vi "GoopDebugger.vi"(1 "ClassToOpen":string, 5 "error in (no error)":errorcluster) -> (19 "error out":errorcluster)   [LabVIEW 2020]
uses:
  <resource>/Framework/Providers/Open_GDS/SubVIs/GOOP_HelpButton.ctl
  <resource>/Framework/Providers/Open_GDS/ClassProviders/Common/LvClass_class/GDSLvClass_ProviderTypes.ctl
  <vilib>/Utility/miscctls.llb/LVRectTypeDef.ctl
  <resource>/Framework/Providers/Open_GDS/ClassProviders/Provider_EndevoGOOP300/ClassWriterGOOP300_class/ClassWriterGOOP300.lvclass
panel:
  in  "_GOOP4Control":bool
  in  "_Help":bool
  in  "_HelpDebugger":T1
  in  "_AttributeType":bool
  in  "_Classes":u16(ring) caption="Classes" items=["View all objects", "-", "GA.lvclass", "GB.lvclass", "GC.lvclass", "GD.lvclass", "File.lvclass", "MyFile.lvclass", "-", "Refresh list"]
  in  "_KillObject":bool
  in  "SortName":bool
  in  "SortId":bool
  out "_NoOfObjects":i32 caption="No of objects"
  in  "_Objects":i32(listbox) caption="Objects"
  out "_Project":string caption="Project"
  in  "_KillAll":bool
  in  "Next":bool
  in  "Prev":bool
  out "AttributeType":string
  in  "_LockPanel":bool
  in  "Update":bool
  in  "_Action":T2(ring) caption="Action"
  out "_Size (kB)":dbl caption="Size (kB)" format="%#.1f"
  out "_Locked?":bool caption="Locked"
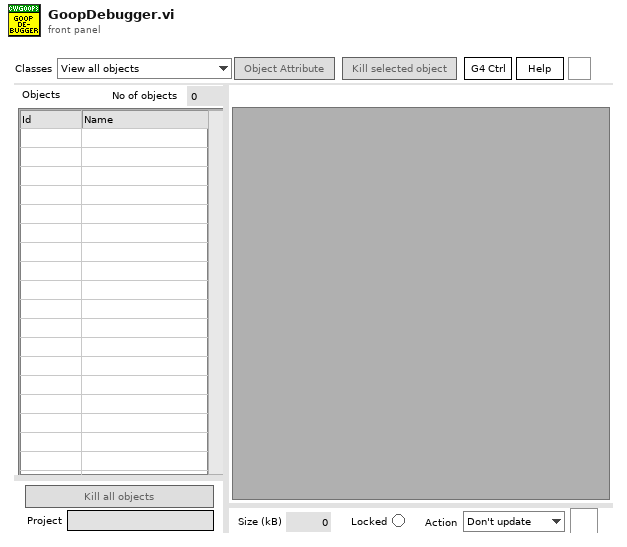
[diagram p1: front panel]
types:
  T1 = typedef "GOOP_HelpButton.ctl" = bool
  T2 = enum16{"Don't update", "Update once", "10ms", "100ms", "500ms", "1s", "2s", "Modify"}
  T3 = typedef "GDSLvClass_ProviderTypes.ctl" = enum16{"UnKnown(LabVOOP)", "Native", "EndevoGOOP3", "OpenG(RootObject)", "OpenG(OpenG_Object)", "EndevoGOOP4", "JKI1"}
  T4 = cluster{"Ref":i32, "Class":string, "Name":string, "ClassProvider":T3}[]
  T5 = typedef "LVRectTypeDef.ctl" = cluster{"Left":i16, "Top":i16, "Right":i16, "Bottom":i16}
  T6 = cluster{"Front Panel.WinBounds":T5, "FP.Behavior":enum32{"Invalid", "Default", "Floating", "Floating/Auto-Hide", "Modal"}}
  T7 = cluster{"DebugQueue":refnum<queue>, "Classes":string[], "ClassAttribute":bool, "NoClassesFound":bool, "ObjRefs":refnum<vi>[], "ClassAttRefs":refnum<vi>[], "ObjStatus":refnum<vi>[], "CurrentClassViewing":string, "ClassAttributeViewing":bool, "OldAction":enum16{"Don't update", "Update once", "10ms", "100ms", "500ms", "1s", "2s", "Modify"}, "ObjectAttString":string, "ClassAttString":string, "KillAllStr":string, "KillTheseStr":string, "IdSort":bool, "MyComputerRef":refnum<vi>, "ClassType":T3[], "ClRefs":refnum<vi>[], "ParentObjeRefs":refnum<vi>[], "G4GetObjStatusRef":refnum<vi>, "G4ParentClasses":string[], "G4AttLevel":i32, "G4NewAttribute":bool, "G4AttRefs":refnum<vi>, "Objects":cluster{"Refs":variant, "VI Name":string, "Object name":string, "ClassProvider":T3}[], "PrevoiusG4AttLevel":i32, "Application":refnum<vi>, "G4ClassAttRefs":refnum<vi>}
  T8 = enum32{"Invalid", "Default", "Floating", "Floating/Auto-Hide", "Modal"}
  T9 = cluster{"Refs":variant, "VI Name":string, "Object name":string, "ClassProvider":T3}[]
  T10 = enum8{"Enabled", "Disabled", "Disabled and Grayed Out"}
  T11 = cluster{"Object names":string[], "Refs":variant[], "ObjectAttributeLocked":bool, "ClassAttributeLocked":bool, "ObjAttribute":variant, "ClassAttribute":variant}
  T12 = cluster{"Refs":variant, "VI Name":string, "Object name":string, "ClassProvider":T3}
  T13 = cluster{i32, cluster{"Refs":variant, "VI Name":string, "Object name":string, "ClassProvider":T3}, "Item Names":string[]}
  T14 = cluster{i32, cluster{"Refs":variant, "VI Name":string, "Object name":string, "ClassProvider":T3}, "Item Names":string[]}[]
  T15 = cluster{"VI Name":string, cluster{"Refs":variant, "VI Name":string, "Object name":string, "ClassProvider":T3}, "Item Names":string[]}
  T16 = cluster{"VI Name":string, cluster{"Refs":variant, "VI Name":string, "Object name":string, "ClassProvider":T3}, "Item Names":string[]}[]
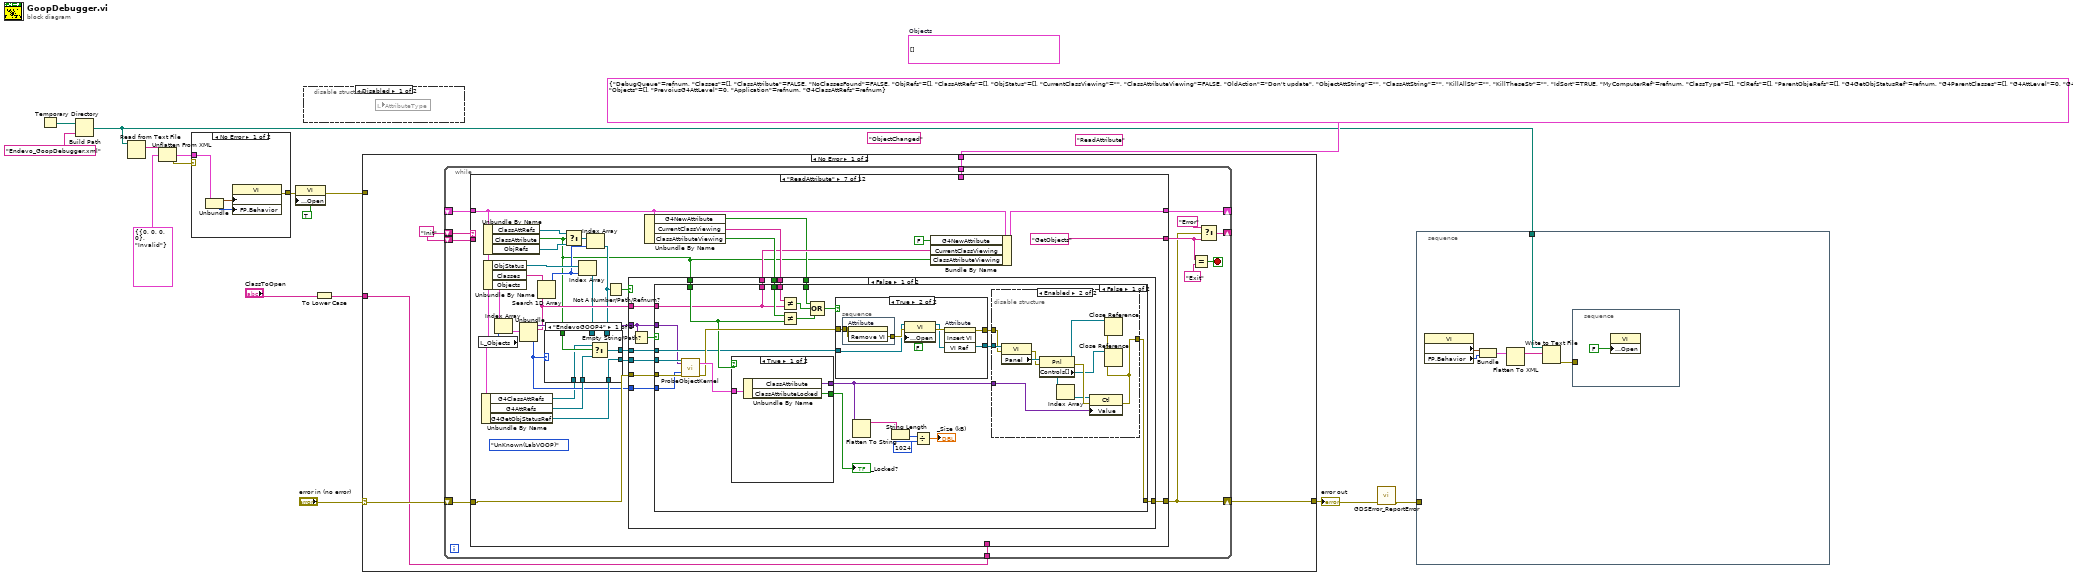
[diagram p0: block diagram]
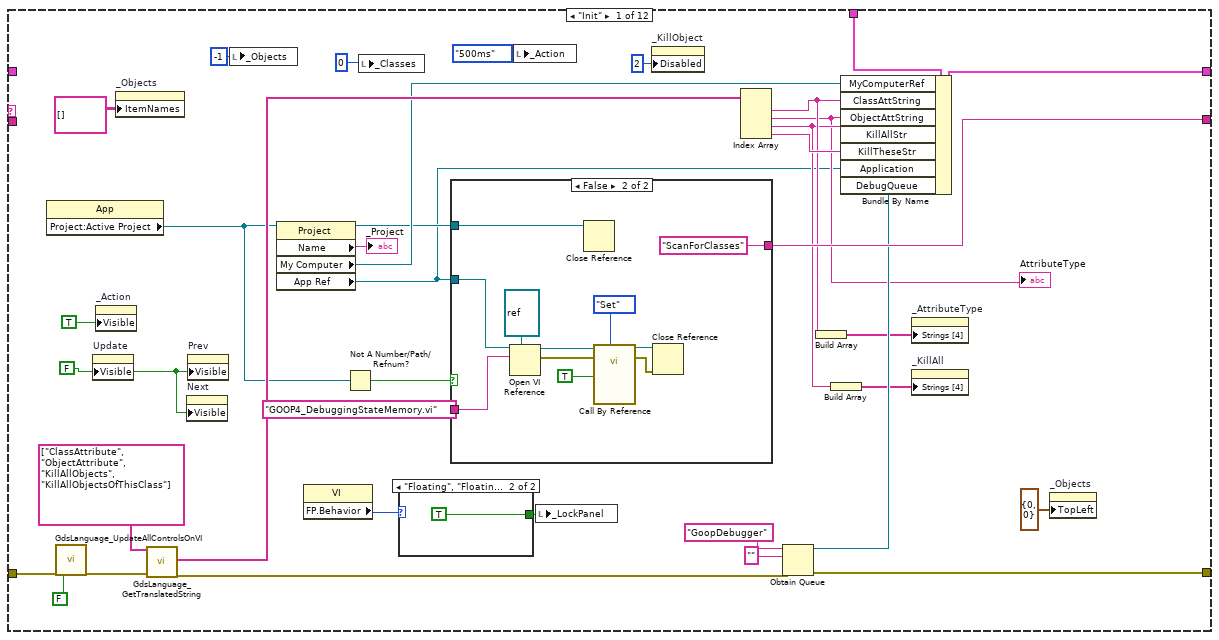
[diagram p4: hidden frame]
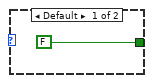
[diagram p5: hidden frame]
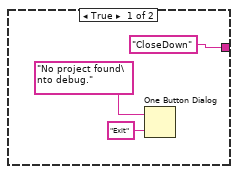
[diagram p6: hidden frame]
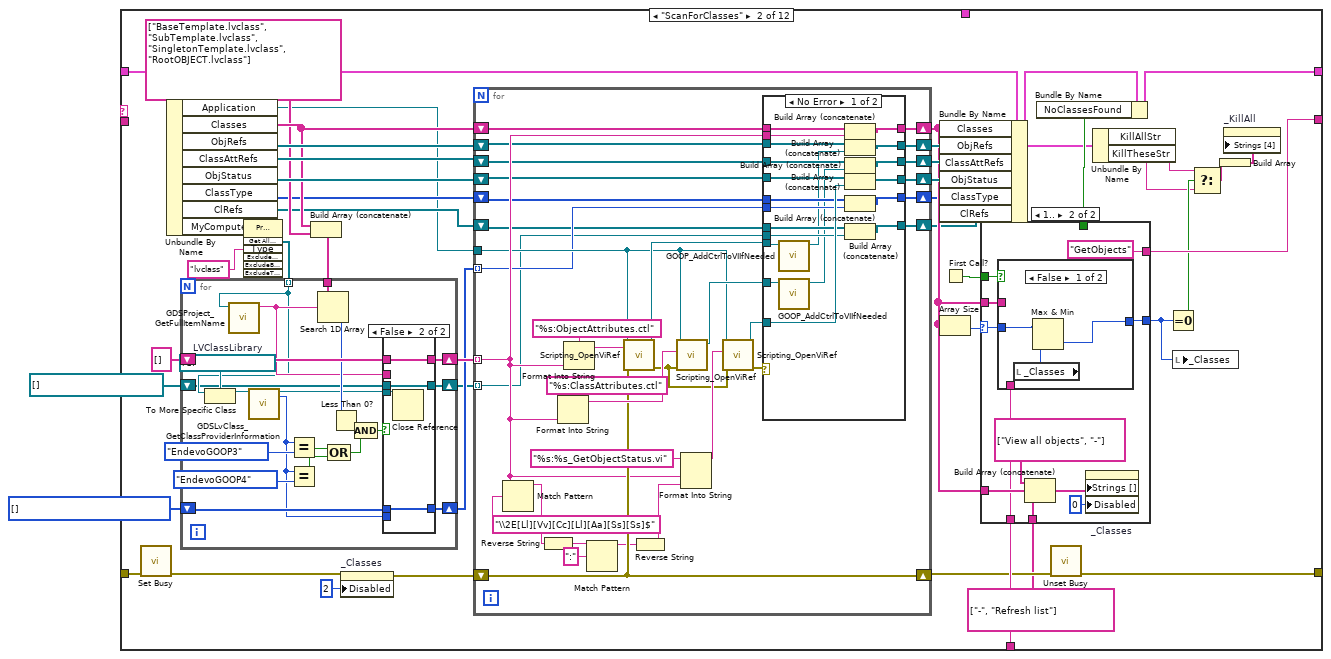
[diagram p7: hidden frame]
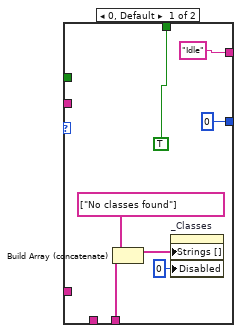
[diagram p8: hidden frame]
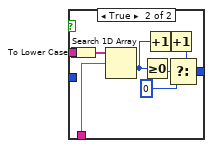
[diagram p9: hidden frame]
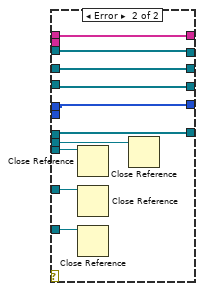
[diagram p10: hidden frame]
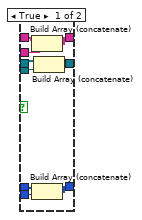
[diagram p11: hidden frame]
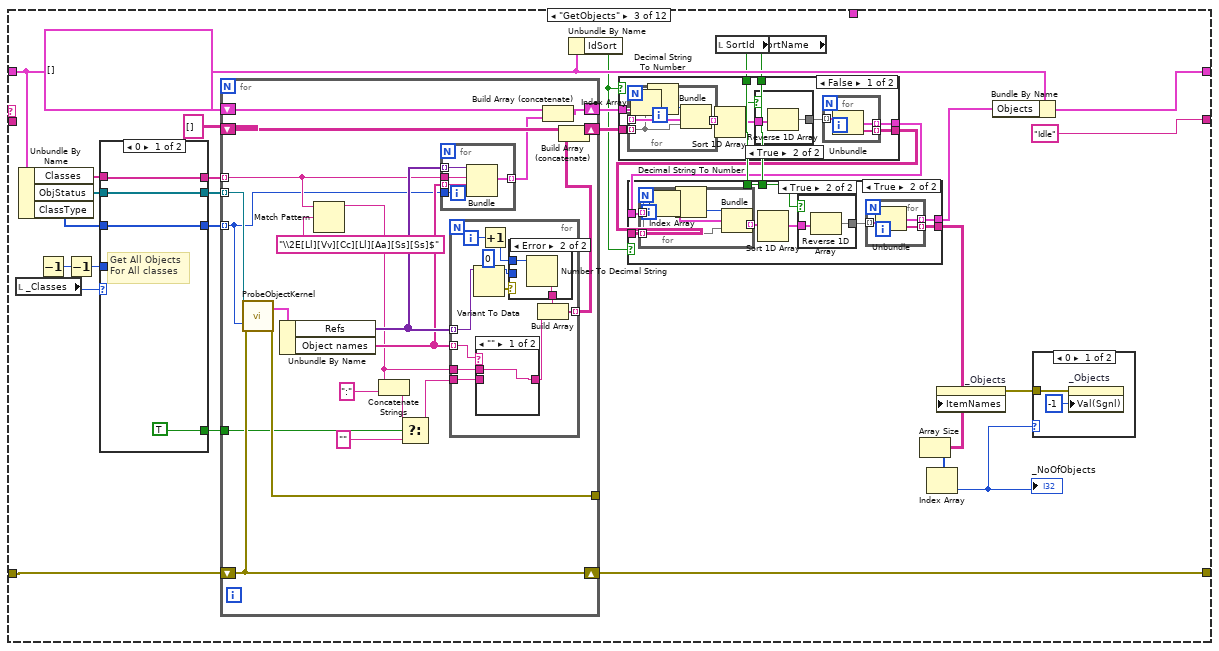
[diagram p12: hidden frame]
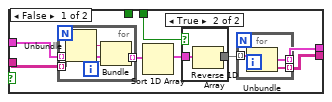
[diagram p13: hidden frame]
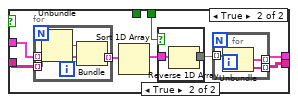
[diagram p17: hidden frame]
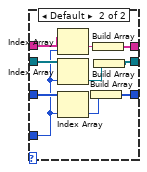
[diagram p20: hidden frame]
diagram:
  (unwired) "ObjectChanged"
  (unwired) T4 []  # Objects
  (unwired) "ReadAttribute"
  n1 = Temporary Directory() -> (w10:path)
  n2 = Build Path(base path=w10, name or relative path="Endevo_GoopDebugger.xml") -> (appended path=w9:path)
  n3 = Read from Text File(file (use dialog)=w9) -> (text=w8:string)  [unwired: 3 in, 3 out]
  n4 = Unflatten From XML(xml string=w8, type=T6 {"Front Panel.WinBounds"={"Left"=0, "Top"=0, "Right"=0, "Bottom"=0}, "FP.Behavior"=enum."Invalid"} ("cluster")) -> (value=w5:T6, error out=w4:errorcluster)  [unwired: 1 in]
  n5 = case shown="No Error" w4 {
    tunnel: [w20 _] -> w6
    tunnel: w5 -> [w19 _]
    frame No Error {
      n6 = Unbundle(w19) -> ("Front Panel.WinBounds"=w18:T5, "FP.Behavior"=w17:T8)
      n7 = property class="VI"("Front Panel.WinBounds"=w18, "FP.Behavior"=w17) -> (error out=w20:errorcluster)  [unwired: 2 in, 1 out]
    }
    frame Error {
    }
  }
  n8 = property class="VI"(error in=w6, "Front Panel.Open"=TRUE ("Front Panel Window:Open")) -> (error out=w3:errorcluster)  [unwired: 1 in, 1 out]
  n9 = disable-structure shown="Disabled" {
    frame Disabled {
      n10 = local read "AttributeType"() -> ()  [unwired: 1 in]
    }
    frame Enabled {
    }
  }
  n11 = To Lower Case(string="ClassToOpen") -> (all lower case string=w1:string)
  n12 = case shown="No Error" "error in (no error)" {
    selector: "error in (no error)" -> [w25 w1029]
    tunnel: [w24 w1029] -> w13
    tunnel: T7 {"DebugQueue"=refnum, "Classes"=[], "ClassAttribute"=FALSE, "NoClassesFound"=FALSE, "ObjRefs"=[], "ClassAttRefs"=[], "ObjStatus"=[], "CurrentClassViewing"="", "ClassAttributeViewing"=FALSE, "OldAction"=enum."Don't update", "ObjectAttString"="", "ClassAttString"="", "KillAllStr"="", "KillTheseStr"="", "IdSort"=TRUE, "MyComputerRef"=refnum, "ClassType"=[], "ClRefs"=[], "ParentObjeRefs"=[], "G4GetObjStatusRef"=refnum, "G4ParentClasses"=[], "G4AttLevel"=0, "G4NewAttribute"=FALSE, "G4AttRefs"=refnum, "Objects"=[], "PrevoiusG4AttLevel"=0, "Application"=refnum, "G4ClassAttRefs"=refnum} ("output cluster") -> [w23 _]
    tunnel: w1 -> [w21 _]
    tunnel: w3 -> [_ _]
    frame No Error {
      w22 = "Init"
      n13 = while {
        shift-right: [w28] -> w24
        shift-left: w25 -> [w38]
        shift-right: [w33] -> _
        shift-left: w22 -> [w29]
        shift-right: [w36] -> _
        shift-left: _ -> [w37]
        tunnel: w23 -> [w31]
        shift-left: w22 -> [w27]
        tunnel: w21 -> [w26]
        stop <- w34 stop-if-true
        n14 = case shown="\"ReadAttribute\"" w29 {
          selector: w29 -> [_ _ _ _ _ _ _ _ _ _ _ w1016]
          tunnel: w37 -> [_ w134 w276 w431 w574 w635 w740 w864 w959 w984 w1012 w1017]
          tunnel: [w74 w116 w285 w432 w573 w648 w747 w863 w959 w984 w1012 w1017] -> w36
          tunnel: w38 -> [w63 w113 w291 w435 w576 w646 w760 w877 w957 w973 w1013 _]
          tunnel: [w49 w110 w290 w435 w576 w645 w761 w878 w955 w974 w1013 errorcluster {"status"=FALSE, "code"=0, "source"=""} ("error IO")] -> w28
          tunnel: [w66 w125 "Idle" w436 "ReadAttribute" "ReadAttribute" "GetObjects" "GetObjects" "GetObjects" "GetObjects" "Idle" w1018] -> w30
          tunnel: w31 -> [w56 _ _ _ _ _ _ _ _ _ _ _]
          tunnel: w27 -> [_ _ _ _ _ _ _ _ _ _ _ w1015]
          tunnel: w26 -> [_ w119 _ _ _ _ _ _ _ _ _ _]
          frame "Init" {
            w41 = FALSE ("Visible")
            n15 = property class="App"() -> ("Project:Active Project"=w47:refnum<vi>)  [unwired: 2 in, 2 out]
            n16 = call <resource>:"GdsLanguage_UpdateAllControlsOnVI.vi"("error in (no error)"=w63, "CreateLanguageFile(Use this to create a languageFile)"=FALSE) -> ("error out"=w61:errorcluster)  [unwired: 16 in, 1 out]
            n17 = property on="Update" class="Bool"("Visible"=w41) -> ()  [unwired: 2 in, 2 out]
            n18 = property on="_Action" class="Enum (strict)"("Visible"=TRUE) -> ()  [unwired: 2 in, 2 out]
            n19 = property on="_Objects" class="MCListbox (strict)"("ItemNames"=string[][] [] ("Item Names")) -> ()  [unwired: 2 in, 2 out]
            n20 = call <resource>:"GdsLanguage_GetTranslatedString.vi"("StringID(s)"=string[] ["ClassAttribute", "ObjectAttribute", "KillAllObjects", "KillAllObjectsOfThisClass"] ("Strings [4]"), "error in (no error)"=w61) -> ("StringsOut"=w58:string[], "error out"=w60:errorcluster)  [unwired: 14 in, 2 out]
            n21 = property on="Next" class="Bool"("Visible"=w41) -> ()  [unwired: 2 in, 2 out]
            n22 = property on="Prev" class="Bool"("Visible"=w41) -> ()  [unwired: 2 in, 2 out]
            n23 = local write "_Objects"(-1 ("Objects")) -> ()
            n24 = property class="Project"(reference=w47) -> (reference out=w44:refnum<vi>, "Name"=→"_Project":string, "My Computer"=w45:refnum<vi>, "App Ref"=w39:refnum<vi>)  [unwired: 1 in, 1 out]
            n25 = property class="VI"() -> ("FP.Behavior"=w65:T8)  [unwired: 2 in, 2 out]
            n26 = Not A Number/Path/Refnum?(number/path/refnum=w47) -> (NaN/Path/Refnum?=w46:bool)
            n27 = local write "_Classes"(0) -> ()
            n28 = case shown="\"Floating\", \"Floating/Auto-Hide\"" w65 {
              tunnel: [FALSE ("LockPanel") TRUE ("LockPanel")] -> w64
              frame Default {
              }
              frame "Floating", "Floating/Auto-Hide" {
              }
            }
            n29 = case shown="False" w46 {
              tunnel: ["CloseDown" "ScanForClasses"] -> w66
              tunnel: w44 -> [_ w89]
              tunnel: w39 -> [_ w81]
              tunnel: "GOOP4_DebuggingStateMemory.vi" -> [_ w80]
              frame True {
                n30 = One Button Dialog(message="No project found\nto debug.", button name ("OK")="Exit") -> ()  [unwired: 1 out]
              }
              frame False {
                n31 = Open VI Reference(type specifier VI Refnum (for type only)=refnum<vi> refnum, application reference (local)=w81, vi path=w80) -> (vi reference=w87:refnum<vi>, error out=w88:errorcluster)  [unwired: 3 in]
                n32 = Close Reference(reference=w89) -> ()  [unwired: 1 in, 1 out]
                n33 = call-by-ref "?"(reference=w87, error in=w88, "Action(Read)"=enum16{"Read", "Set"}."Set", "DebuggingStateIn"=TRUE) -> (reference out=w86:refnum<vi>, error out=w85:errorcluster)  [unwired: 8 in, 2 out]
                n34 = Close Reference(reference=w86, error in (no error)=w85) -> ()  [unwired: 1 out]
              }
            }
            n35 = local write "_Action"(T2."500ms" ("Action")) -> ()
            n36 = local write "_LockPanel"(w64) -> ()
            n37 = property on="_KillObject" class="Bool"("Disabled"=u8 2) -> ()  [unwired: 2 in, 2 out]
            n38 = Index Array(array=w58) -> (element #1=w54:string, element #2=w42:string, element #3=w52:string, element #4=w55:string)  [unwired: 4 in]
            "AttributeType" <- w42
            n39 = Obtain Queue(name (unnamed)="GoopDebugger", element data type="", error in (no error)=w60) -> (queue out=w57:refnum<queue>, error out=w49:errorcluster)  [unwired: 2 in, 1 out]
            n40 = Build Array(w54) -> (w53:string[])
            n41 = Build Array(w52) -> (w51:string[])
            n42 = Bundle By Name(cluster=w56, "MyComputerRef"=w45, "ClassAttString"=w54, "ObjectAttString"=w42, "KillAllStr"=w52, "KillTheseStr"=w55, "Application"=w39, "DebugQueue"=w57) -> (w74:T7)
            n43 = property on="_AttributeType" class="Bool"("Strings [4]"=w53) -> ()  [unwired: 2 in, 2 out]
            n44 = property on="_KillAll" class="Bool"("Strings [4]"=w51) -> ()  [unwired: 2 in, 2 out]
            n45 = property on="_Objects" class="MCListbox (strict)"("TopLeft"=cluster{"Row":u32, "Column":u32} {"Row"=0, "Column"=0} ("Top Left Visible Cell")) -> ()  [unwired: 2 in, 2 out]
          }
          frame "ScanForClasses" {
            w98 = T3[] [] items=["UnKnown(LabVOOP)", "Native", "EndevoGOOP3", "OpenG(RootObject)", "OpenG(OpenG_Object)", "EndevoGOOP4", "JKI1"]
            n46 = call <vilib>:"Set Busy.vi"("error in (no error)"=w113) -> ("error out"=w112:errorcluster)  [unwired: 9 in, 1 out]
            n47 = Unbundle By Name(w134) -> ("Application"=w91:refnum<vi>, "Classes"=w123:string[], "ObjRefs"=w132:refnum<vi>[], "ClassAttRefs"=w131:refnum<vi>[], "ObjStatus"=w130:refnum<vi>[], "ClassType"=w93:T3[], "ClRefs"=w92:refnum<vi>[], "MyComputerRef"=w101:refnum<vi>)
            n48 = invoke class="ProjectItem" method="Get All Descendents"(reference=w101, "Type"="lvclass") -> ("All Descendents"=w117:refnum<vi>[])  [unwired: 5 in, 6 out]
            n49 = Build Array (concatenate)(w123, string[] ["BaseTemplate.lvclass", "SubTemplate.lvclass", "SingletonTemplate.lvclass", "RootOBJECT.lvclass"] ("array")) -> (w122:string[])
            n50 = for {
              shift-right: [w249] -> w133
              shift-left: string[] [] -> [w250]
              tunnel: w122 -> [w247]
              tunnel: w117 -> [w236] mode=indexing
              shift-right: [w233] -> w99
              shift-left: w98 -> [w235]
              shift-right: [w231] -> w96
              shift-left: refnum<vi>[] [] -> [w230]
              w244 = refnum<vi> refnum  # LVClassLibrary
              n51 = To More Specific Class(target class=w244, reference=w236) -> (specific class reference=w238:refnum<vi>)  [unwired: 1 in, 1 out]
              n52 = call <resource>:"GDSProject_GetFullItemName.vi"("ProjectItem Refnum"=w236) -> ("ItemFullName"=w237:string)  [unwired: 5 in, 1 out]
              n53 = call <resource>:"GDSLvClass_GetClassProviderInformation.vi"("Class Refnum In"=w238) -> ("Class Refnum Out"=w232:refnum<vi>, "ClassProvider"=w234:T3)  [unwired: 16 in, 1 out]
              n54 = Equal?(x=w234, y=GDSLvClass_ProviderTypes."EndevoGOOP3") -> (x = y?=w243:bool)
              n55 = Equal?(x=w234, y=GDSLvClass_ProviderTypes."EndevoGOOP4") -> (x = y?=w242:bool)
              n56 = Search 1D Array(1D array=w247, element=w237) -> (index of element=w246:i32)  [unwired: 1 in]
              n57 = Compound Arithmetic op=OR(w243, w242) -> (w241:bool)
              n58 = Less Than 0?(x=w246) -> (x < 0?=w245:bool)
              n59 = Compound Arithmetic op=AND(w245, w241) -> (w248:bool)
              n60 = case shown="False" w248 {
                tunnel: w250 -> [w259 w263]
                tunnel: [w258 w263] -> w249
                tunnel: w237 -> [w257 _]
                tunnel: w235 -> [w256 w262]
                tunnel: w234 -> [w255 _]
                tunnel: [w254 w262] -> w233
                tunnel: w232 -> [w253 w261]
                tunnel: [w252 w260] -> w231
                tunnel: w230 -> [w251 w260]
                frame True {
                  n61 = Build Array (concatenate)(w259, w257) -> (w258:string[])
                  n62 = Build Array (concatenate)(w256, w255) -> (w254:T3[])
                  n63 = Build Array (concatenate)(w251, w253) -> (w252:refnum<vi>[])
                }
                frame False {
                  n64 = Close Reference(reference=w261) -> ()  [unwired: 1 in, 1 out]
                }
              }
            }
            n65 = property on="_Classes" class="Ring (strict)"(error in=w112, "Disabled"=u8 2) -> (error out=w115:errorcluster)  [unwired: 1 in, 1 out]
            n66 = for {
              shift-right: [w192] -> w111
              shift-left: w115 -> [w192]
              tunnel: w133 -> [w189] mode=indexing
              shift-right: [w190] -> w120
              shift-left: w123 -> [w191]
              shift-right: [w185] -> w129
              shift-left: w132 -> [w188]
              shift-right: [w184] -> w128
              shift-left: w131 -> [w187]
              shift-right: [w183] -> w127
              shift-left: w130 -> [w186]
              tunnel: w91 -> [w179]
              shift-right: [w170] -> w97
              shift-left: w93 -> [w171]
              tunnel: w99 -> [w169] mode=indexing
              shift-right: [w168] -> w95
              shift-left: w92 -> [w167]
              tunnel: w96 -> [w166] mode=indexing
              n67 = Match Pattern(string=w189, regular expression="\\2E[Ll][Vv][Cc][Ll][Aa][Ss][Ss]$") -> (before substring=w175:string)  [unwired: 1 in, 3 out]
              n68 = Reverse String(1:w175) -> (0:w178:string)
              n69 = Format Into String(format string="%s:ClassAttributes.ctl", w189) -> (resulting string=w196:string)  [unwired: 2 in, 1 out]
              n70 = Format Into String(format string="%s:ObjectAttributes.ctl", w189) -> (resulting string=w198:string)  [unwired: 2 in, 1 out]
              n71 = Match Pattern(string=w178, regular expression=":") -> (before substring=w176:string)  [unwired: 1 in, 3 out]
              n72 = call <resource>:"Scripting_OpenViRef.vi"("error in"=w192, "ViPath/ViName/Viref"=w198, "AppRef"=w179) -> ("error out"=w173:errorcluster, "vi reference"=w182:refnum<vi>)  [unwired: 6 in, 1 out]
              n73 = Reverse String(1:w176) -> (0:w174:string)
              n74 = call <resource>:"Scripting_OpenViRef.vi"("error in"=w173, "ViPath/ViName/Viref"=w196, "AppRef"=w179) -> ("vi reference"=w181:refnum<vi>)  [unwired: 6 in, 2 out]
              n75 = Format Into String(format string="%s:%s_GetObjectStatus.vi", w189, w174) -> (resulting string=w193:string)  [unwired: 2 in, 1 out]
              n76 = call <resource>:"Scripting_OpenViRef.vi"("error in"=w173, "ViPath/ViName/Viref"=w193, "AppRef"=w179) -> ("error out"=w172:errorcluster, "vi reference"=w180:refnum<vi>)  [unwired: 6 in, 1 out]
              n77 = case shown="No Error" w172 {
                tunnel: w191 -> [w219 w229]
                tunnel: [w218 w229] -> w190
                tunnel: w189 -> [w217 _]
                tunnel: w188 -> [w216 w228]
                tunnel: w187 -> [w215 w227]
                tunnel: w186 -> [w214 w226]
                tunnel: [w213 w228] -> w185
                tunnel: [w212 w227] -> w184
                tunnel: [w211 w226] -> w183
                tunnel: w182 -> [w201 w225]
                tunnel: w181 -> [w203 w224]
                tunnel: w180 -> [w210 w223]
                tunnel: w171 -> [w209 w222]
                tunnel: [w208 w222] -> w170
                tunnel: w169 -> [w207 _]
                tunnel: [w206 w220] -> w168
                tunnel: w167 -> [w205 w220]
                tunnel: w166 -> [w204 w221]
                frame No Error {
                  n78 = call <resource>:"GOOP_AddCtrlToVIIfNeeded.vi"("Ctrl VI in"=w201) -> ("VI out"=w200:refnum<vi>)  [unwired: 8 in, 2 out]
                  n79 = call <resource>:"GOOP_AddCtrlToVIIfNeeded.vi"("Ctrl VI in"=w203) -> ("VI out"=w202:refnum<vi>)  [unwired: 8 in, 2 out]
                  n80 = Build Array (concatenate)(w219, w217) -> (w218:string[])
                  n81 = Build Array (concatenate)(w216, w200) -> (w213:refnum<vi>[])
                  n82 = Build Array (concatenate)(w215, w202) -> (w212:refnum<vi>[])
                  n83 = Build Array (concatenate)(w214, w210) -> (w211:refnum<vi>[])
                  n84 = Build Array (concatenate)(w209, w207) -> (w208:T3[])
                  n85 = Build Array (concatenate)(w205, w204) -> (w206:refnum<vi>[])
                }
                frame Error {
                  n86 = Close Reference(reference=w225) -> ()  [unwired: 1 in, 1 out]
                  n87 = Close Reference(reference=w224) -> ()  [unwired: 1 in, 1 out]
                  n88 = Close Reference(reference=w223) -> ()  [unwired: 1 in, 1 out]
                  n89 = Close Reference(reference=w221) -> ()  [unwired: 1 in, 1 out]
                }
              }
            }
            n90 = Bundle By Name(cluster=w134, "Classes"=w120, "ObjRefs"=w129, "ClassAttRefs"=w128, "ObjStatus"=w127, "ClassType"=w97, "ClRefs"=w95) -> (w103:T7)
            n91 = Array Size(array=w120) -> (size(s)=w126:i32)
            n92 = First Call?() -> (First Call?: T/F=w121:bool)
            n93 = case shown="1.." w126 {
              selector: w126 -> [_ w151]
              tunnel: [TRUE _] -> w124
              tunnel: ["Idle" "GetObjects"] -> w125
              tunnel: w120 -> [_ w150]
              tunnel: w121 -> [_ w148]
              tunnel: w120 -> [_ w147]
              tunnel: w119 -> [_ w146]
              tunnel: string[] ["-", "Refresh list"] ("Strings []") -> [w138 w144]
              tunnel: [0 w143] -> w102
              frame 0, Default {
                n94 = Build Array (concatenate)(string[] ["No classes found"] ("Strings []"), w138) -> (w137:string[])
                n95 = property on="_Classes" class="Ring (strict)"("Strings []"=w137, "Disabled"=u8 0) -> ()  [unwired: 2 in, 2 out]
              }
              frame 1.. {
                n96 = case shown="False" w148 {
                  tunnel: [w155 w159] -> w143
                  tunnel: w151 -> [w154 _]
                  tunnel: w147 -> [_ w165]
                  tunnel: w146 -> [_ w164]
                  frame False {
                    n97 = local read "_Classes"() -> (w156:u16)
                    n98 = Max & Min(x=w154, y=w156) -> (min(x,y)=w155:i32)  [unwired: 1 out]
                  }
                  frame True {
                    n99 = To Lower Case(string=w165) -> (all lower case string=w163:string[])
                    n100 = Search 1D Array(1D array=w163, element=w164) -> (index of element=w160:i32)  [unwired: 1 in]
                    n101 = Greater Or Equal To 0?(x=w160) -> (x >= 0?=w161:bool)
                    n102 = Increment(x=w160) -> (x+1=w162:i32)
                    n103 = Increment(x=w162) -> (x+1=w158:i32)
                    n104 = Select(t=w158, s=w161, f=0) -> (s? t:f=w159:i32)
                  }
                }
                n105 = Build Array (concatenate)(string[] ["View all objects", "-"] ("array"), w150, w144) -> (w153:string[])
                n106 = property on="_Classes" class="Ring (strict)"("Strings []"=w153, "Disabled"=u8 0) -> ()  [unwired: 2 in, 2 out]
              }
            }
            n107 = Bundle By Name(cluster=w103, "NoClassesFound"=w124) -> (w116:T7)
            n108 = call <vilib>:"Unset Busy.vi"("error in (no error)"=w111) -> ("error out"=w110:errorcluster)  [unwired: 10 in]
            n109 = Unbundle By Name(w103) -> ("KillAllStr"=w106:string, "KillTheseStr"=w105:string)
            n110 = Equal To 0?(x=w102) -> (x = 0?=w108:bool)
            n111 = local write "_Classes"(w102) -> ()
            n112 = Select(t=w106, s=w108, f=w105) -> (s? t:f=w107:string)
            n113 = Build Array(w107) -> (w104:string[])
            n114 = property on="_KillAll" class="Bool"("Strings [4]"=w104) -> ()  [unwired: 2 in, 2 out]
          }
          frame "GetObjects" {
            n115 = local read "_Classes"() -> (w283:u16)
            n116 = Unbundle By Name(w276) -> ("Classes"=w284:string[], "ObjStatus"=w289:refnum<vi>[], "ClassType"=w266:T3[])
            n117 = Decrement(x=w283) -> (x-1=w267:u16)
            n118 = Decrement(x=w267) -> (x-1=w268:u16)
            n119 = case shown="0" w283 {
              tunnel: w284 -> [w372 w382]
              tunnel: w289 -> [w371 w381]
              tunnel: w268 -> [_ w375]
              tunnel: [w372 w378] -> w288
              tunnel: [w371 w377] -> w287
              tunnel: [TRUE _] -> w282
              tunnel: w266 -> [w369 w376]
              tunnel: [w369 w373] -> w265
              frame 0 {
                # "Get All Objects\nFor All classes"
              }
              frame Default {
                n120 = Index Array(array=w382, index=w375) -> (element=w380:string)
                n121 = Index Array(array=w381, index=w375) -> (element=w379:refnum<vi>)
                n122 = Index Array(array=w376, index=w375) -> (element=w374:T3)
                n123 = Build Array(w374) -> (w373:T3[])
                n124 = Build Array(w380) -> (w378:string[])
                n125 = Build Array(w379) -> (w377:refnum<vi>[])
              }
            }
            n126 = for {
              tunnel: w287 -> [w403] mode=indexing
              tunnel: w288 -> [w391] mode=indexing
              shift-right: [w394] -> w290
              shift-left: w291 -> [w394]
              shift-right: [w400] -> w277
              shift-left: string[][] [] ("Item Names") -> [w401]
              shift-right: [w398] -> w278
              shift-left: T9 [] -> [w399]
              tunnel: [w393] -> _
              tunnel: w282 -> [w390]
              tunnel: w265 -> [w384] mode=indexing
              n127 = call <resource>:"ProbeObjectKernel.vi"("ObjectStatus"=w403, "ClassProvider"=w384, "error in"=w394) -> ("DebuggerOut"=w402:T11, "error out"=w393:errorcluster)  [unwired: 15 in]
              n128 = Unbundle By Name(w402) -> ("Refs"=w397:variant[], "Object names"=w396:string[])
              n129 = Match Pattern(string=w391, regular expression="\\2E[Ll][Vv][Cc][Ll][Aa][Ss][Ss]$") -> (before substring=w385:string)  [unwired: 1 in, 3 out]
              n130 = Concatenate Strings(w385, ":" ("string")) -> (w386:string)
              n131 = Select(t=w386, s=w390, f="") -> (s? t:f=w389:string)
              n132 = for {
                tunnel: w397 -> [w408] mode=indexing
                tunnel: w391 -> [w407]
                tunnel: w396 -> [w406] mode=indexing
                tunnel: [w405] -> w395 mode=indexing
                tunnel: w384 -> [w404]
                n133 = Bundle("Refs"=w408, "VI Name"=w407, "Object name"=w406, "ClassProvider"=w404) -> (w405:T12)  [unwired: 1 in]
              }
              n134 = for {
                tunnel: w397 -> [w414] mode=indexing
                tunnel: w396 -> [w418] mode=indexing
                tunnel: [w419] -> w383 mode=indexing
                tunnel: w389 -> [w417]
                tunnel: w385 -> [w415]
                i -> [w410]
                n135 = Variant To Data(type=0 ("input 1"), Variant=w414) -> (data=w412:i32, error out=w411:errorcluster)  [unwired: 1 in]
                n136 = case shown="\"\"" w418 {
                  selector: w418 -> [_ w429]
                  tunnel: w417 -> [_ w428]
                  tunnel: [w426 w427] -> w416
                  tunnel: w415 -> [w426 _]
                  frame "" {
                  }
                  frame Default {
                    n137 = Format Into String(format string="%s", initial string=w428, w429) -> (resulting string=w427:string)  [unwired: 1 in, 1 out]
                  }
                }
                n138 = Increment(x=w410) -> (x+1=w409:i32)
                n139 = case shown="Error" w411 {
                  tunnel: [w422 w425] -> w420
                  tunnel: w412 -> [w421 _]
                  tunnel: w409 -> [_ w424]
                  frame No Error {
                    n140 = Format Into String(format string="%08x", w421) -> (resulting string=w422:string)  [unwired: 2 in, 1 out]
                  }
                  frame Error {
                    n141 = Number To Decimal String(number=w424) -> (decimal integer string=w425:string)  [unwired: 1 in]
                  }
                }
                n142 = Build Array(w420, w416) -> (w419:string[])
              }
              n143 = Build Array (concatenate)(w399, w395) -> (w398:T9)
              n144 = Build Array (concatenate)(w401, w383) -> (w400:string[][])
            }
            n145 = Unbundle By Name(w276) -> ("IdSort"=w273:bool)
            n146 = local read "SortId"() -> (w275:bool)
            n147 = local read "SortName"() -> (w274:bool)
            n148 = case shown="False" w273 {
              tunnel: w278 -> [w336 w353]
              tunnel: w275 -> [w335 _]
              tunnel: w277 -> [w332 w352]
              tunnel: [w331 w351] -> w271
              tunnel: [w330 w350] -> w272
              tunnel: w274 -> [_ w349]
              frame False {
                n149 = for {
                  tunnel: w336 -> [w348] mode=indexing
                  tunnel: w332 -> [w346] mode=indexing
                  tunnel: [w347] -> w337 mode=indexing
                  n150 = Index Array(array=w346) -> (element=w345:string)  [unwired: 1 in]
                  n151 = Decimal String To Number(string=w345) -> (number=w344:i32)  [unwired: 2 in, 1 out]
                  n152 = Bundle(w344, w348, "Item Names"=w346) -> (w347:T13)  [unwired: 1 in]
                }
                n153 = Sort 1D Array(array=w337) -> (sorted array=w334:T14)
                n154 = case shown="True" w335 {
                  tunnel: w334 -> [w338 w340]
                  tunnel: [w338 w339] -> w333
                  frame False {
                  }
                  frame True {
                    n155 = Reverse 1D Array(array=w340) -> (reversed array=w339:T14)
                  }
                }
                n156 = for {
                  tunnel: w333 -> [w343] mode=indexing
                  tunnel: [w342] -> w331 mode=indexing
                  tunnel: [w341] -> w330 mode=indexing
                  n157 = Unbundle(w343) -> (w342:T12, "Item Names"=w341:string[])  [unwired: 1 out]
                }
              }
              frame True {
                n158 = for {
                  tunnel: w353 -> [w364] mode=indexing
                  tunnel: w352 -> [w366] mode=indexing
                  tunnel: [w365] -> w354 mode=indexing
                  n159 = Unbundle(w364) -> ("VI Name"=w363:string)  [unwired: 3 out]
                  n160 = Bundle("VI Name"=w363, w364, "Item Names"=w366) -> (w365:T15)  [unwired: 1 in]
                }
                n161 = Sort 1D Array(array=w354) -> (sorted array=w355:T16)
                n162 = case shown="True" w349 {
                  tunnel: w355 -> [w357 w359]
                  tunnel: [w357 w358] -> w356
                  frame False {
                  }
                  frame True {
                    n163 = Reverse 1D Array(array=w359) -> (reversed array=w358:T16)
                  }
                }
                n164 = for {
                  tunnel: w356 -> [w362] mode=indexing
                  tunnel: [w361] -> w351 mode=indexing
                  tunnel: [w360] -> w350 mode=indexing
                  n165 = Unbundle(w362) -> (w361:T12, "Item Names"=w360:string[])  [unwired: 1 out]
                }
              }
            }
            n166 = case shown="True" w273 {
              tunnel: w271 -> [w297 w317]
              tunnel: w275 -> [_ w316]
              tunnel: w272 -> [w296 w313]
              tunnel: [w295 w312] -> w270
              tunnel: w274 -> [w294 _]
              tunnel: [w293 w311] -> w269
              frame False {
                n167 = for {
                  tunnel: w297 -> [w308] mode=indexing
                  tunnel: w296 -> [w310] mode=indexing
                  tunnel: [w309] -> w298 mode=indexing
                  n168 = Unbundle(w308) -> ("VI Name"=w307:string)  [unwired: 3 out]
                  n169 = Bundle("VI Name"=w307, w308, "Item Names"=w310) -> (w309:T15)  [unwired: 1 in]
                }
                n170 = Sort 1D Array(array=w298) -> (sorted array=w299:T16)
                n171 = case shown="True" w294 {
                  tunnel: w299 -> [w301 w303]
                  tunnel: [w301 w302] -> w300
                  frame False {
                  }
                  frame True {
                    n172 = Reverse 1D Array(array=w303) -> (reversed array=w302:T16)
                  }
                }
                n173 = for {
                  tunnel: w300 -> [w306] mode=indexing
                  tunnel: [w305] -> w295 mode=indexing
                  tunnel: [w304] -> w293 mode=indexing
                  n174 = Unbundle(w306) -> (w305:T12, "Item Names"=w304:string[])  [unwired: 1 out]
                }
              }
              frame True {
                n175 = for {
                  tunnel: w317 -> [w327] mode=indexing
                  tunnel: w313 -> [w328] mode=indexing
                  tunnel: [w329] -> w318 mode=indexing
                  n176 = Index Array(array=w328) -> (element=w326:string)  [unwired: 1 in]
                  n177 = Decimal String To Number(string=w326) -> (number=w325:i32)  [unwired: 2 in, 1 out]
                  n178 = Bundle(w325, w327, "Item Names"=w328) -> (w329:T13)  [unwired: 1 in]
                }
                n179 = Sort 1D Array(array=w318) -> (sorted array=w315:T14)
                n180 = case shown="True" w316 {
                  tunnel: w315 -> [w319 w321]
                  tunnel: [w319 w320] -> w314
                  frame False {
                  }
                  frame True {
                    n181 = Reverse 1D Array(array=w321) -> (reversed array=w320:T14)
                  }
                }
                n182 = for {
                  tunnel: w314 -> [w324] mode=indexing
                  tunnel: [w323] -> w312 mode=indexing
                  tunnel: [w322] -> w311 mode=indexing
                  n183 = Unbundle(w324) -> (w323:T12, "Item Names"=w322:string[])  [unwired: 1 out]
                }
              }
            }
            n184 = Array Size(array=w269) -> (size(s)=w281:i32[])
            n185 = Index Array(array=w281) -> (element=w279:i32)  [unwired: 1 in]
            "_NoOfObjects" <- w279
            n186 = property on="_Objects" class="MCListbox (strict)"("ItemNames"=w269) -> (error out=w280:errorcluster)  [unwired: 2 in, 1 out]
            n187 = Bundle By Name(cluster=w276, "Objects"=w270) -> (w285:T7)
            n188 = case shown="0" w279 {
              tunnel: w280 -> [w368 _]
              frame 0 {
                n189 = property on="_Objects" class="MCListbox (strict)"(error in=w368, "Val(Sgnl)"=-1 ("Value (Signaling)")) -> ()  [unwired: 1 in, 2 out]
              }
              frame Default {
              }
            }
          }
          frame "Idle" {
            n190 = Unbundle By Name(w431) -> ("NoClassesFound"=w433:bool)
            n191 = case shown="True" w433 {
              tunnel: [w450 5000] -> w434
              frame False {
                n192 = property on="_Objects" class="MCListbox (strict)"() -> ("ItemNames"=w444:string[][])  [unwired: 2 in, 2 out]
                n193 = Array Size(array=w444) -> (size(s)=w443:i32[])
                n194 = local read "_Objects"() -> (w449:i32)
                n195 = Index Array(array=w443) -> (element=w442:i32)  [unwired: 1 in]
                n196 = Greater Than 0?(x=w442) -> (x > 0?=w439:bool)
                n197 = Greater Or Equal To 0?(x=w449) -> (x >= 0?=w441:bool)
                n198 = local read "_Action"() -> (w451:T2)
                n199 = And(x=w439, y=w441) -> (x .and. y?=w440:bool)
                n200 = Select(t=u8 0 ("Disabled"), s=w440, f=u8 2) -> (s? t:f=w437:u8)
                n201 = Select(t=u8 0 ("Disabled"), s=w439, f=u8 2) -> (s? t:f=w438:u8)
                n202 = case shown="\"10ms\"" w451 {
                  tunnel: [-1 10 100 500 1000 2000] -> w450
                  frame Default {
                  }
                  frame "10ms" {
                  }
                  frame "100ms" {
                  }
                  frame "500ms" {
                  }
                  frame "1s" {
                  }
                  frame "2s" {
                  }
                }
                n203 = property on="_KillObject" class="Bool"("Disabled"=w437) -> ()  [unwired: 2 in, 2 out]
                n204 = property on="_AttributeType" class="Bool"("Disabled"=w437) -> ()  [unwired: 2 in, 2 out]
                n205 = property on="_KillAll" class="Bool"("Disabled"=w438) -> ()  [unwired: 2 in, 2 out]
              }
              frame True {
                w459 = u8 2 ("Disabled")
                n206 = property on="_KillAll" class="Bool"("Disabled"=w459) -> ()  [unwired: 2 in, 2 out]
                n207 = property on="_AttributeType" class="Bool"("Disabled"=w459) -> ()  [unwired: 2 in, 2 out]
                n208 = property on="_KillObject" class="Bool"("Disabled"=w459) -> ()  [unwired: 2 in, 2 out]
              }
            }
            n209 = event shown="[7] \"_Objects\": Value Change" {
              selector: _ -> [_ _ _ _ _ _ _ _ _ _ _ _ _ _ _ _ _]
              dyn-events: _ -> [_ _ _ _ _ _ _ _ _ _ _ _ _ _ _ _ _]
              timeout: w434 -> [_ _ _ _ _ _ _ _ _ _ _ _ _ _ _ _ _]
              tunnel: [w467 w472 "UpdateAttribute" "KillObject" "Idle" "KillObject" "ObjectChanged" w512 "Idle" "UpdatePreNext" "UpdatePreNext" "CloseDown" "GetObjects" "GetObjects" w550 "Idle" "Idle"] -> w436
              tunnel: w433 -> [w468 _ _ _ _ _ _ _ _ _ _ _ _ _ _ _ _]
              tunnel: w431 -> [w465 w471 w483 w487 w491 w495 w508 w510 w523 w529 w535 w537 w542 w546 w561 w568 w569]
              tunnel: [w465 w470 w483 w487 w491 w495 w507 w509 w523 w528 w534 w537 w541 w545 w561 w568 w569] -> w432
              tunnel: w431 -> [_ _ w482 _ _ _ w502 _ _ w527 w533 _ _ _ w558 _ _]
              event Timeout {
                n210 = event-data() -> ()  [unwired: 1 in, 1 out]
                n211 = local read "_Objects"() -> (w464:i32)
                n212 = Greater Or Equal To 0?(x=w464) -> (x >= 0?=w463:bool)
                n213 = Select(t="ReadAttribute", s=w463, f="GetObjects") -> (s? t:f=w461:string)
                n214 = Select(t="ScanForClasses", s=w468, f=w461) -> (s? t:f=w467:string)
              }
              event "_Action": Value Change {
                n215 = event-data() -> ("OldVal"=w469:T2)  [unwired: 1 in]
                n216 = case shown="\"Update once\"" "_Action" {
                  tunnel: ["Idle" "ReadAttribute" "ReadAttribute" "PrepareToModify"] -> w472
                  frame "Don't update" {
                  }
                  frame Default {
                  }
                  frame "Update once" {
                    n217 = local write "_Action"(T2."Don't update" ("Action")) -> ()
                  }
                  frame "Modify" {
                    n218 = property on="Update" class="Bool"("Visible"=TRUE) -> ()  [unwired: 2 in, 2 out]
                    n219 = property on="_Action" class="Enum (strict)"("Visible"=FALSE) -> ()  [unwired: 2 in, 2 out]
                  }
                }
                n220 = Bundle By Name(cluster=w471, "OldAction"=w469) -> (w470:T7)
              }
              event "Update": Value Change {
                n221 = event-data() -> ()  [unwired: 1 in, 1 out]
                n222 = Unbundle By Name(w482) -> ("OldAction"=w481:T2)
                n223 = local write "_Action"(w481) -> ()
                n224 = property on="Update" class="Bool"("Visible"=FALSE) -> ()  [unwired: 2 in, 2 out]
                n225 = property on="_Action" class="Enum (strict)"("Visible"=TRUE) -> ()  [unwired: 2 in, 2 out]
              }
              event "_KillObject": Value Change {
                n226 = event-data() -> ()  [unwired: 1 in, 4 out]
              }
              event "_LockPanel": Value Change {
                n227 = event-data() -> ()  [unwired: 1 in, 1 out]
                n228 = property class="VI"() -> ("FP.Behavior"=w490:T8)  [unwired: 2 in, 2 out]
                n229 = case shown="Default" w490 {
                  tunnel: [T8."Floating" ("Front Panel Window:Behavior") T8."Default" ("Front Panel Window:Behavior")] -> w489
                  frame Default {
                  }
                  frame "Floating", "Floating/Auto-Hide" {
                  }
                }
                n230 = property class="VI"("FP.Behavior"=w489) -> ()  [unwired: 2 in, 2 out]
              }
              event "_KillAll": Value Change {
                n231 = event-data() -> ()  [unwired: 1 in, 4 out]
                n232 = local write "_Objects"(-1 ("Objects")) -> ()
              }
              event "_AttributeType": Value Change {
                n233 = event-data() -> ()  [unwired: 1 in, 1 out]
                n234 = Unbundle By Name(w502) -> ("ClassAttString"=w499:string, "ObjectAttString"=w500:string)
                n235 = Unbundle By Name(w502) -> ("ClassAttribute"=w503:bool)
                n236 = Not(x=w503) -> (.not. x?=w504:bool)
                n237 = Select(t=w499, s=w503, f=w500) -> (s? t:f=w506:string)
                n238 = Select(t=w500, s=w503, f=w499) -> (s? t:f=w498:string)
                n239 = Build Array(w506) -> (w501:string[])
                n240 = local write "AttributeType"(w498) -> ()
                n241 = property on="_AttributeType" class="Bool"("Strings [4]"=w501) -> ()  [unwired: 2 in, 2 out]
                n242 = Bundle By Name(cluster=w508, "ClassAttribute"=w504) -> (w507:T7)
              }
              event "_Objects": Value Change {
                n243 = event-data() -> ()  [unwired: 1 in, 1 out]
                n244 = case shown="-1" "_Objects" {
                  tunnel: ["ObjectChanged" "Idle"] -> w512
                  tunnel: [_ u8 2 ("Disabled")] -> w511
                  tunnel: w510 -> [w514 w520]
                  tunnel: [w514 w519] -> w509
                  frame 0, Default {
                  }
                  frame -1 {
                    w516 = FALSE
                    w517 = T10."Disabled and Grayed Out" ("Disabled")
                    n245 = invoke on="Attribute" class="SubPanel" method="Remove VI"() -> ()  [unwired: 3 in, 3 out]
                    n246 = Bundle By Name(cluster=w520, "CurrentClassViewing"="") -> (w519:T7)
                    n247 = property on="Prev" class="Bool"("DisabledEnum"=w517) -> ()  [unwired: 2 in, 2 out]
                    n248 = property on="Prev" class="Bool"("Visible"=w516) -> ()  [unwired: 2 in, 2 out]
                    n249 = property on="Next" class="Bool"("DisabledEnum"=w517) -> ()  [unwired: 2 in, 2 out]
                    n250 = property on="Next" class="Bool"("Visible"=w516) -> ()  [unwired: 2 in, 2 out]
                  }
                }
                n251 = property on="_KillObject" class="Bool"("Disabled"=w511) -> ()  [unwired: 2 in, 2 out]
              }
              event "_GOOP4Control": Value Change {
                n252 = event-data() -> ()  [unwired: 1 in, 1 out]
                n253 = call <resource>:"GOOP_StartDebuggerController.vi"() -> ()  [unwired: 19 in, 1 out]
              }
              event "Next": Value Change {
                n254 = event-data() -> ()  [unwired: 1 in, 1 out]
                n255 = Unbundle By Name(w527) -> ("G4AttLevel"=w525:i32)
                n256 = Increment(x=w525) -> (x+1=w526:i32)
                n257 = Bundle By Name(cluster=w529, "PrevoiusG4AttLevel"=w525, "G4AttLevel"=w526) -> (w528:T7)
              }
              event "Prev": Value Change {
                n258 = event-data() -> ()  [unwired: 1 in, 1 out]
                n259 = Unbundle By Name(w533) -> ("G4AttLevel"=w532:i32)
                n260 = Decrement(x=w532) -> (x-1=w531:i32)
                n261 = Bundle By Name(cluster=w535, "G4AttLevel"=w531) -> (w534:T7)
              }
              event Panel Close? {
                n262 = event-data() -> ()  [unwired: 1 in, 4 out]
                n263 = event-data("Discard?"=TRUE) -> ()  [unwired: 1 in, 1 out]
              }
              event "SortId": Value Change {
                n264 = event-data() -> ()  [unwired: 1 in, 1 out]
                n265 = Bundle By Name(cluster=w542, "IdSort"=TRUE) -> (w541:T7)
              }
              event "SortName": Value Change {
                n266 = event-data() -> ()  [unwired: 1 in, 1 out]
                n267 = Bundle By Name(cluster=w546, "IdSort"=FALSE) -> (w545:T7)
              }
              event "_Classes": Value Change {
                n268 = event-data() -> ()  [unwired: 1 in, 2 out]
                n269 = property on="_Classes" class="Ring (strict)"() -> ("Strings []"=w554:string[])  [unwired: 2 in, 2 out]
                n270 = Unbundle By Name(w558) -> ("KillAllStr"=w557:string, "KillTheseStr"=w556:string)
                n271 = Array Size(array=w554) -> (size(s)=w551:i32)
                n272 = Increment(x="_Classes") -> (x+1=w552:u16)
                n273 = Equal To 0?(x="_Classes") -> (x = 0?=w560:bool)
                n274 = Greater Or Equal?(x=w552, y=w551) -> (x >= y?=w549:bool)
                n275 = case shown="True" w549 {
                  tunnel: ["GetObjects" "ScanForClasses"] -> w550
                  frame False {
                  }
                  frame True {
                    w563 = u16 0 items=["View all objects", "-", "MyBaseClass.lvclass", "MySub1.lvclass", "Sub2.lvclass", "Base1.lvclass", "-", "Refresh list"] ("_Classes")
                    n276 = local write "_Classes"(w563) -> ()
                  }
                }
                n277 = Select(t=w557, s=w560, f=w556) -> (s? t:f=w559:string)
                n278 = Build Array(w559) -> (w555:string[])
                n279 = property on="_Objects" class="MCListbox (strict)"("TopLeft"=cluster{"Row":u32, "Column":u32} {"Row"=0, "Column"=0} ("Top Left Visible Cell")) -> ()  [unwired: 2 in, 2 out]
                n280 = property on="_KillAll" class="Bool"("Strings [4]"=w555) -> ()  [unwired: 2 in, 2 out]
              }
              event Value Change {
                n281 = event-data() -> ()  [unwired: 1 in, 3 out]
                n282 = fn#1354() -> (1:w566:bool)  [unwired: 1 out]
                n283 = Not(x=w566) -> (.not. x?=w565:bool)
                n284 = Control Help Window(1:w565) -> ()  [unwired: 1 in]
              }
              event "_Help": Value Change {
                n285 = event-data() -> ()  [unwired: 1 in, 3 out]
                n286 = call <resource>:"GOOP_HelpMain.vi"() -> ()  [unwired: 12 in]
              }
            }
          }
          frame "ObjectChanged" {
            (unwired) GDSLvClass_ProviderTypes."UnKnown(LabVOOP)" ("ClassProvider")
            n287 = Unbundle By Name(w574) -> ("ClRefs"=w577:refnum<vi>[], "Classes"=w579:string[], "Objects"=w581:T9)
            n288 = local read "_Objects"() -> (w575:i32)
            n289 = Index Array(array=w581, index=w575) -> (element=w580:T12)
            n290 = Unbundle(w580) -> ("VI Name"=w578:string, "ClassProvider"=w572:T3)  [unwired: 2 out]
            n291 = case shown="\"EndevoGOOP4\"" w572 {
              tunnel: w579 -> [_ w614]
              tunnel: w578 -> [_ w598]
              tunnel: w577 -> [_ w613]
              tunnel: w574 -> [_ w590]
              tunnel: w575 -> [_ _]
              tunnel: w574 -> [w584 w603]
              tunnel: [w584 w602] -> w573
              tunnel: [FALSE TRUE] -> w571
              frame Default {
              }
              frame "EndevoGOOP4" {
                n292 = Unbundle By Name(w590) -> ("ObjRefs"=w596:refnum<vi>[], "ClassAttRefs"=w587:refnum<vi>[])
                n293 = Unbundle By Name(w590) -> ("ObjStatus"=w604:refnum<vi>[])
                n294 = Search 1D Array(1D array=w614, element=w598) -> (index of element=w586:i32)  [unwired: 1 in]
                n295 = Index Array(array=w613, index=w586) -> (element=w612:refnum<vi>)
                n296 = while {
                  shift-right: [w615] -> _
                  shift-left: w612 -> [w618]
                  shift-right: [w616] -> w600
                  shift-left: string[] [] -> [w619]
                  tunnel: [w617] -> w609
                  i -> [w617]
                  stop <- w620 stop-if-true
                  n297 = property class="LVClassLibrary"(reference=w618) -> ("Parent"=w615:refnum<vi>)  [unwired: 1 in, 2 out]
                  n298 = Not A Number/Path/Refnum?(number/path/refnum=w615) -> (NaN/Path/Refnum?=w620:bool)
                  n299 = case shown="False" w620 {
                    tunnel: [w624 w626] -> w616
                    tunnel: w619 -> [w625 w626]
                    tunnel: w615 -> [w623 _]
                    frame False {
                      n300 = property class="LVClassLibrary"(reference=w623) -> ("Name"=w622:string)  [unwired: 1 in, 2 out]
                      n301 = Build Array (concatenate)(w625, w622) -> (w624:string[])
                    }
                    frame True {
                    }
                  }
                  n302 = case shown="Default" w617 {
                    tunnel: w618 -> [w621 _]
                    tunnel: w616 -> [_ _]
                    frame Default {
                      n303 = Close Reference(reference=w621) -> ()  [unwired: 1 in, 1 out]
                    }
                    frame 0 {
                    }
                  }
                }
                n304 = Index Array(array=w604, index=w586) -> (element=w601:refnum<vi>)
                n305 = Index Array(array=w596, index=w586) -> (element=w595:refnum<vi>)
                n306 = Index Array(array=w587, index=w586) -> (element=w585:refnum<vi>)
                n307 = Greater Than 0?(x=w609) -> (x > 0?=w608:bool)
                n308 = Unbundle By Name(w590) -> ("ClassAttribute"=w592:bool)
                n309 = Select(t=T10."Enabled" ("Disabled"), s=w608, f=T10."Disabled and Grayed Out" ("Disabled")) -> (s? t:f=w605:T10)
                n310 = Select(t="Class Attribute, %s" ("format string"), s=w592, f="Object Attribute, %s" ("format string")) -> (s? t:f=w588:string)
                n311 = property on="Next" class="Bool"("DisabledEnum"=w605) -> ()  [unwired: 2 in, 2 out]
                n312 = property on="Prev" class="Bool"("DisabledEnum"=T10."Disabled and Grayed Out" ("Disabled")) -> ()  [unwired: 2 in, 2 out]
                n313 = Format Into String(format string=w588, w598) -> (resulting string=w599:string)  [unwired: 2 in, 1 out]
                n314 = Bundle By Name(cluster=w603, "G4NewAttribute"=TRUE, "G4AttLevel"=-1, "G4ParentClasses"=w600, "G4GetObjStatusRef"=w601, "G4AttRefs"=w595, "G4ClassAttRefs"=w585) -> (w602:T7)
                n315 = local write "AttributeType"(w599) -> ()
              }
            }
            n316 = property on="Next" class="Bool"("Visible"=w571) -> ()  [unwired: 2 in, 2 out]
            n317 = property on="Prev" class="Bool"("Visible"=w571) -> ()  [unwired: 2 in, 2 out]
          }
          frame "UpdatePreNext" {
            n318 = Unbundle By Name(w635) -> ("Application"=w633:refnum<vi>, "G4ParentClasses"=w651:string[], "G4AttLevel"=w650:i32)
            n319 = Unbundle By Name(w635) -> ("Classes"=w640:string[], "Objects"=w639:T9)
            n320 = local read "_Objects"() -> (w637:i32)
            n321 = Index Array(array=w639, index=w637) -> (element=w638:T12)
            n322 = Unbundle(w638) -> ("VI Name"=w636:string)  [unwired: 3 out]
            n323 = Search 1D Array(1D array=w640, element=w636) -> (index of element=w634:i32)  [unwired: 1 in]
            n324 = case shown="Default" w650 {
              selector: w650 -> [w691 _]
              tunnel: w651 -> [w693 _]
              tunnel: [w673 w730] -> w649
              tunnel: w646 -> [w676 w729]
              tunnel: [w676 w729] -> w645
              tunnel: [w671 w723] -> w643
              tunnel: w635 -> [w664 w725]
              tunnel: [w661 w722] -> w641
              tunnel: w636 -> [w660 w722]
              tunnel: w635 -> [w663 w721]
              tunnel: [w662 w721] -> w631
              tunnel: w634 -> [w658 w719]
              tunnel: w633 -> [w652 _]
              tunnel: [w656 w718] -> w632
              frame Default {
                w669 = T10."Enabled" ("Disabled")
                n325 = Array Size(array=w693) -> (size(s)=w692:i32)
                n326 = Increment(x=w691) -> (x+1=w690:i32)
                n327 = Index Array(array=w693, index=w691) -> (element=w654:string)
                n328 = Equal?(x=w692, y=w690) -> (x = y?=w688:bool)
                n329 = Match Pattern(string=w654, regular expression="\\2E[Ll][Vv][Cc][Ll][Aa][Ss][Ss]$") -> (before substring=w682:string)  [unwired: 1 in, 3 out]
                n330 = Format Into String(format string="%s:ObjectAttributes.ctl", w654) -> (resulting string=w678:string)  [unwired: 2 in, 1 out]
                n331 = Format Into String(format string="%s:ClassAttributes.ctl", w654) -> (resulting string=w653:string)  [unwired: 2 in, 1 out]
                n332 = Reverse String(1:w682) -> (0:w685:string)
                n333 = Unbundle By Name(w664) -> ("ObjStatus"=w667:refnum<vi>[])
                n334 = Unbundle By Name(w664) -> ("ObjRefs"=w668:refnum<vi>[])
                n335 = Unbundle By Name(w664) -> ("ClassAttRefs"=w659:refnum<vi>[])
                n336 = Select(t=T10."Disabled and Grayed Out" ("Disabled"), s=w688, f=w669) -> (s? t:f=w670:T10)
                n337 = Match Pattern(string=w685, regular expression=":") -> (before substring=w683:string)  [unwired: 1 in, 3 out]
                n338 = Reverse String(1:w683) -> (0:w681:string)
                n339 = Format Into String(format string="%s:%s_GetObjectStatus.vi", w654, w681) -> (resulting string=w680:string)  [unwired: 2 in, 1 out]
                n340 = Index Array(array=w668, index=w658) -> (element=w665:refnum<vi>)
                n341 = Index Array(array=w659, index=w658) -> (element=w657:refnum<vi>)
                n342 = Index Array(array=w667, index=w658) -> (element=w666:refnum<vi>)
                n343 = call <resource>:"Scripting_OpenViRef.vi"("error in"=w676, "ViPath/ViName/Viref"=w680, "AppRef"=w652) -> ("error out"=w677:errorcluster, "vi reference"=w674:refnum<vi>)  [unwired: 6 in, 1 out]
                n344 = call <resource>:"Scripting_OpenViRef.vi"("error in"=w677, "ViPath/ViName/Viref"=w678, "AppRef"=w652) -> ("error out"=w675:errorcluster, "vi reference"=w672:refnum<vi>)  [unwired: 6 in, 1 out]
                n345 = case shown="No Error" w675 {
                  selector: w675 -> [w700 _]
                  tunnel: w674 -> [w706 _]
                  tunnel: [w706 w714] -> w673
                  tunnel: w672 -> [w705 _]
                  tunnel: [w705 w715] -> w671
                  tunnel: w670 -> [w704 _]
                  tunnel: w669 -> [w703 _]
                  tunnel: w666 -> [_ w714]
                  tunnel: w665 -> [_ w715]
                  tunnel: w663 -> [w702 w717]
                  tunnel: [w702 w716] -> w662
                  tunnel: w654 -> [w701 _]
                  tunnel: [w701 w713] -> w661
                  tunnel: w660 -> [_ w713]
                  tunnel: w657 -> [w695 w709]
                  tunnel: [w696 w709] -> w656
                  tunnel: w653 -> [w699 _]
                  tunnel: w652 -> [w694 _]
                  frame No Error {
                    n346 = call <resource>:"Scripting_OpenViRef.vi"("error in"=w700, "ViPath/ViName/Viref"=w699, "AppRef"=w694) -> ("error out"=w698:errorcluster, "vi reference"=w697:refnum<vi>)  [unwired: 6 in, 1 out]
                    n347 = case shown="Error" w698 {
                      tunnel: w697 -> [w707 _]
                      tunnel: [w707 w708] -> w696
                      tunnel: w695 -> [_ w708]
                      frame No Error {
                      }
                      frame Error {
                      }
                    }
                    n348 = property on="Next" class="Bool"("DisabledEnum"=w704) -> ()  [unwired: 2 in, 2 out]
                    n349 = property on="Prev" class="Bool"("DisabledEnum"=w703) -> ()  [unwired: 2 in, 2 out]
                  }
                  frame Error {
                    n350 = Bundle By Name(cluster=w717, "G4AttLevel"=-1) -> (w716:T7)
                    n351 = property on="Next" class="Bool"("DisabledEnum"=T10."Enabled" ("Disabled")) -> ()  [unwired: 2 in, 2 out]
                    n352 = property on="Prev" class="Bool"("DisabledEnum"=T10."Disabled and Grayed Out" ("Disabled")) -> ()  [unwired: 2 in, 2 out]
                  }
                }
              }
              frame -1 {
                n353 = Unbundle By Name(w725) -> ("ObjRefs"=w726:refnum<vi>[], "ClassAttRefs"=w720:refnum<vi>[])
                n354 = Unbundle By Name(w725) -> ("ObjStatus"=w724:refnum<vi>[])
                n355 = Index Array(array=w726, index=w719) -> (element=w723:refnum<vi>)
                n356 = Index Array(array=w720, index=w719) -> (element=w718:refnum<vi>)
                n357 = Index Array(array=w724, index=w719) -> (element=w730:refnum<vi>)
                n358 = property on="Next" class="Bool"("DisabledEnum"=T10."Enabled" ("Disabled")) -> ()  [unwired: 2 in, 2 out]
                n359 = property on="Prev" class="Bool"("DisabledEnum"=T10."Disabled and Grayed Out" ("Disabled")) -> ()  [unwired: 2 in, 2 out]
              }
            }
            n360 = Unbundle By Name(w631) -> ("ClassAttribute"=w630:bool)
            n361 = Select(t="Class Attribute, %s" ("format string"), s=w630, f="Object Attribute, %s" ("format string")) -> (s? t:f=w627:string)
            n362 = Format Into String(format string=w627, w641) -> (resulting string=w642:string)  [unwired: 2 in, 1 out]
            n363 = Bundle By Name(cluster=w631, "G4NewAttribute"=TRUE, "G4GetObjStatusRef"=w649, "G4AttRefs"=w643, "G4ClassAttRefs"=w632) -> (w648:T7)
            n364 = local write "AttributeType"(w642) -> ()
          }
          frame "ReadAttribute" {
            (unwired) GDSLvClass_ProviderTypes."UnKnown(LabVOOP)" ("ClassProvider")
            n365 = local read "_Objects"() -> (w759:i32)
            n366 = Unbundle By Name(w740) -> ("G4ClassAttRefs"=w731:refnum<vi>, "G4AttRefs"=w734:refnum<vi>, "G4GetObjStatusRef"=w739:refnum<vi>)
            n367 = Unbundle By Name(w740) -> ("ObjStatus"=w754:refnum<vi>[], "Classes"=w755:string[], "Objects"=w758:T9)
            n368 = Unbundle By Name(w740) -> ("ClassAttRefs"=w752:refnum<vi>[], "ClassAttribute"=w732:bool, "ObjRefs"=w753:refnum<vi>[])
            n369 = Index Array(array=w758, index=w759) -> (element=w757:T12)
            n370 = Unbundle(w757) -> ("Refs"=w756:variant, "VI Name"=w749:string, "ClassProvider"=w733:T3)  [unwired: 1 out]
            n371 = Search 1D Array(1D array=w755, element=w749) -> (index of element=w745:i32)  [unwired: 1 in]
            n372 = Select(t=w752, s=w732, f=w753) -> (s? t:f=w751:refnum<vi>[])
            n373 = Index Array(array=w754, index=w745) -> (element=w742:refnum<vi>)
            n374 = Index Array(array=w751, index=w745) -> (element=w738:refnum<vi>)
            n375 = case shown="\"EndevoGOOP4\"" w733 {
              tunnel: [w766 w768] -> w741
              tunnel: w742 -> [_ w768]
              tunnel: w739 -> [w766 _]
              tunnel: [w763 w767] -> w737
              tunnel: w738 -> [_ w767]
              tunnel: w734 -> [w764 _]
              tunnel: w732 -> [w765 _]
              tunnel: w731 -> [w762 _]
              frame "EndevoGOOP4" {
                n376 = Select(t=w762, s=w765, f=w764) -> (s? t:f=w763:refnum<vi>)
              }
              frame Default {
              }
            }
            n377 = Not A Number/Path/Refnum?(number/path/refnum=w738) -> (NaN/Path/Refnum?=w743:bool)
            n378 = Unbundle By Name(w740) -> ("G4NewAttribute"=w735:bool, "CurrentClassViewing"=w750:string, "ClassAttributeViewing"=w748:bool)
            n379 = case shown="False" w743 {
              tunnel: [w781 w854] -> w761
              tunnel: w760 -> [w780 w854]
              tunnel: w756 -> [w769 _]
              tunnel: w750 -> [w779 _]
              tunnel: w749 -> [w778 _]
              tunnel: w748 -> [w777 _]
              tunnel: [w776 _] -> w746
              tunnel: w732 -> [w775 _]
              tunnel: w741 -> [w774 _]
              tunnel: w737 -> [w773 _]
              tunnel: w735 -> [w772 _]
              tunnel: w733 -> [w771 _]
              frame False {
                n380 = Empty String/Path?(string/path=w769) -> (empty?=w770:bool)
                n381 = case shown="False" w770 {
                  tunnel: [w790 w853] -> w781
                  tunnel: w780 -> [w802 w853]
                  tunnel: w775 -> [w795 _]
                  tunnel: w779 -> [w797 _]
                  tunnel: w778 -> [w792 _]
                  tunnel: w777 -> [w796 _]
                  tunnel: [w792 _] -> w776
                  tunnel: w774 -> [w787 _]
                  tunnel: w773 -> [w786 _]
                  tunnel: w772 -> [w784 _]
                  tunnel: w771 -> [w783 _]
                  tunnel: w769 -> [w782 _]
                  frame False {
                    n382 = call <resource>:"ProbeObjectKernel.vi"("ObjectStatus"=w787, "Ref"=w782, "ClassProvider"=w783, "error in"=w802) -> ("DebuggerOut"=w803:T11, "error out"=w798:errorcluster)  [unwired: 14 in]
                    n383 = case shown="True" w795 {
                      tunnel: [w849 w852] -> w788
                      tunnel: w803 -> [w848 w851]
                      tunnel: [w847 w850] -> w800
                      frame True {
                        n384 = Unbundle By Name(w848) -> ("ClassAttribute"=w849:variant, "ClassAttributeLocked"=w847:bool)
                      }
                      frame False {
                        n385 = Unbundle By Name(w851) -> ("ObjAttribute"=w852:variant, "ObjectAttributeLocked"=w850:bool)
                      }
                    }
                    "_Locked?" <- w800
                    n386 = Not Equal?(x=w797, y=w792) -> (x != y?=w785:bool)
                    n387 = Not Equal?(x=w796, y=w795) -> (x != y?=w794:bool)
                    n388 = Compound Arithmetic op=OR(w784, w785, w794) -> (w793:bool)
                    n389 = case shown="True" w793 {
                      tunnel: [w838 w843] -> w789
                      tunnel: w798 -> [w838 w842]
                      tunnel: [w837 w839] -> w791
                      tunnel: w786 -> [w837 w840]
                      frame False {
                      }
                      frame True {
                        n390 = stacked-sequence {
                          tunnel: w842 -> [w846]
                          tunnel: [w846] -> w841
                          frame #0 {
                            n391 = invoke on="Attribute" class="SubPanel" method="Remove VI"(error in=w846) -> ()  [unwired: 2 in, 3 out]
                          }
                        }
                        n392 = property class="VI"(reference=w840, error in=w841, "Front Panel.Open"=FALSE ("Front Panel Window:Open")) -> (reference out=w839:refnum<vi>, error out=w844:errorcluster)
                        n393 = invoke on="Attribute" class="SubPanel" method="Insert VI"(error in=w844, "VI Ref"=w839) -> (error out=w843:errorcluster)  [unwired: 2 in, 3 out]
                      }
                    }
                    n394 = Flatten To String(anything=w788) -> (data string=w801:string)  [unwired: 3 in, 2 out]
                    n395 = String Length(string=w801) -> (length=w805:i32)
                    n396 = Divide(x=w805, y=1024) -> (x/y=→"_Size (kB)":dbl)
                    n397 = disable-structure shown="Enabled" {
                      disable-tunnel: w791 -> [w811 w836]
                      disable-tunnel: [w809 w828] -> w790
                      disable-tunnel: w789 -> [w807 w832]
                      disable-tunnel: w788 -> [w806 w831]
                      frame Disabled {
                        n398 = invoke class="VI" method="Ctrl Val.Set"(reference=w811, error in=w807, "Control Name"="Base class", "Value"=w806) -> (reference out=w808:refnum<vi>, error out=w810:errorcluster)  [unwired: 1 in, 3 out]
                        n399 = case shown="Error" w810 {
                          selector: w810 -> [w813 _]
                          tunnel: [w813 w815] -> w809
                          tunnel: w808 -> [_ w820]
                          tunnel: w807 -> [_ w816]
                          tunnel: w806 -> [_ w814]
                          frame No Error {
                          }
                          frame Error {
                            n400 = invoke class="VI" method="Ctrl Val.Set"(reference=w820, error in=w816, "Control Name"="Data", "Value"=w814) -> (reference out=w817:refnum<vi>, error out=w818:errorcluster)  [unwired: 1 in, 3 out]
                            n401 = case shown="Error" w818 {
                              selector: w818 -> [w821 _]
                              tunnel: w817 -> [_ w826]
                              tunnel: w816 -> [_ w825]
                              tunnel: [w821 w824] -> w815
                              tunnel: w814 -> [_ w822]
                              frame No Error {
                              }
                              frame Error {
                                n402 = invoke class="VI" method="Ctrl Val.Set"(reference=w826, error in=w825, "Control Name"="Class attribute", "Value"=w822) -> (error out=w824:errorcluster)  [unwired: 1 in, 4 out]
                              }
                            }
                          }
                        }
                      }
                      frame Enabled {
                        n403 = property class="VI"(reference=w836, error in=w832) -> (error out=w833:errorcluster, "Panel"=w835:refnum<vi>)  [unwired: 1 out]
                        n404 = property class="Pnl"(reference=w835, error in=w833) -> (reference out=w827:refnum<vi>, error out=w834:errorcluster, "Controls[]"=w829:refnum<vi>[])
                        n405 = Index Array(array=w829) -> (element=w830:refnum<vi>)  [unwired: 1 in]
                        n406 = property class="Ctl"(reference=w830, error in=w834, "Value"=w831) -> (error out=w828:errorcluster)  [unwired: 1 out]
                        n407 = Close Reference(reference=w827, error in (no error)=w828) -> ()  [unwired: 1 out]
                        n408 = Close Reference(reference=w829, error in (no error)=w828) -> ()  [unwired: 1 out]
                      }
                    }
                  }
                  frame True {
                    n409 = invoke on="Attribute" class="SubPanel" method="Remove VI"() -> ()  [unwired: 3 in, 3 out]
                  }
                }
              }
              frame True {
                n410 = invoke on="Attribute" class="SubPanel" method="Remove VI"() -> ()  [unwired: 3 in, 3 out]
              }
            }
            n411 = Bundle By Name(cluster=w740, "G4NewAttribute"=FALSE, "CurrentClassViewing"=w746, "ClassAttributeViewing"=w732) -> (w747:T7)
          }
          frame "UpdateAttribute" {
            n412 = Unbundle By Name(w864) -> ("ObjStatus"=w872:refnum<vi>[], "Classes"=w873:string[], "Objects"=w875:T9)
            n413 = Unbundle By Name(w864) -> ("ClassAttRefs"=w869:refnum<vi>[], "ClassAttribute"=w861:bool, "ObjRefs"=w870:refnum<vi>[])
            n414 = local read "_Objects"() -> (w876:i32)
            n415 = Index Array(array=w875, index=w876) -> (element=w874:T12)
            n416 = Unbundle(w874) -> ("Refs"=w855:variant, "VI Name"=w866:string, "ClassProvider"=w857:T3)  [unwired: 1 out]
            n417 = Search 1D Array(1D array=w873, element=w866) -> (index of element=w860:i32)  [unwired: 1 in]
            n418 = Empty String/Path?(string/path=w855) -> (empty?=w856:bool)
            n419 = Select(t=w869, s=w861, f=w870) -> (s? t:f=w868:refnum<vi>[])
            n420 = Index Array(array=w872, index=w860) -> (element=w871:refnum<vi>)
            n421 = Index Array(array=w868, index=w860) -> (element=w859:refnum<vi>)
            n422 = Unbundle By Name(w864) -> ("CurrentClassViewing"=w867:string, "ClassAttributeViewing"=w865:bool)
            n423 = case shown="False" w856 {
              tunnel: [w879 w902] -> w878
              tunnel: w877 -> [w879 w887]
              tunnel: w861 -> [_ w909]
              tunnel: w871 -> [_ w911]
              tunnel: w867 -> [_ w910]
              tunnel: w866 -> [_ w905]
              tunnel: w865 -> [_ w901]
              tunnel: [_ w905] -> w862
              tunnel: w859 -> [_ w904]
              tunnel: w857 -> [_ w896]
              tunnel: w855 -> [_ w895]
              frame True {
                n424 = invoke on="Attribute" class="SubPanel" method="Remove VI"() -> ()  [unwired: 3 in, 3 out]
              }
              frame False {
                n425 = Equal?(x=w910, y=w905) -> (x = y?=w908:bool)
                n426 = Equal?(x=w901, y=w909) -> (x = y?=w907:bool)
                n427 = And(x=w908, y=w907) -> (x .and. y?=w906:bool)
                n428 = case shown="False" w906 {
                  tunnel: [w945 w950] -> w886
                  tunnel: w887 -> [w944 w950]
                  tunnel: [w941 w949] -> w891
                  tunnel: w904 -> [w942 w949]
                  frame False {
                    n429 = stacked-sequence {
                      tunnel: w944 -> [w948]
                      tunnel: [w948] -> w943
                      frame #0 {
                        n430 = invoke on="Attribute" class="SubPanel" method="Remove VI"(error in=w948) -> ()  [unwired: 2 in, 3 out]
                      }
                    }
                    n431 = property class="VI"(reference=w942, error in=w943, "Front Panel.Open"=FALSE ("Front Panel Window:Open")) -> (reference out=w941:refnum<vi>, error out=w946:errorcluster)
                    n432 = invoke on="Attribute" class="SubPanel" method="Insert VI"(error in=w946, "VI Ref"=w941) -> (error out=w945:errorcluster)  [unwired: 2 in, 3 out]
                  }
                  frame True {
                  }
                }
                n433 = property class="VI"(reference=w891, error in=w886) -> (error out=w888:errorcluster, "Panel"=w894:refnum<vi>)  [unwired: 1 out]
                n434 = property class="Pnl"(reference=w894, error in=w888) -> (reference out=w882:refnum<vi>, error out=w889:errorcluster, "Controls[]"=w884:refnum<vi>[])
                n435 = Index Array(array=w884) -> (element=w893:refnum<vi>)  [unwired: 1 in]
                n436 = property class="Ctl"(reference=w893, error in=w889) -> (error out=w885:errorcluster, "Label.Text"=w881:string)  [unwired: 1 out]
                n437 = invoke class="VI" method="Ctrl Val.Get (Deprecated)"(reference=w891, error in=w885, "Control Name"=w881) -> (reference out=w890:refnum<vi>, error out=w892:errorcluster, "Get Control Value"=w880:string)  [unwired: 2 in, 2 out]
                n438 = Close Reference(reference=w884, error in (no error)=w885) -> (error out=w883:errorcluster)
                n439 = case shown="No Error" w892 {
                  selector: w892 -> [w912 _]
                  tunnel: [w912 w919] -> w898
                  tunnel: [w913 w917] -> w897
                  tunnel: w886 -> [_ w915]
                  tunnel: w890 -> [_ w914]
                  tunnel: w880 -> [w913 _]
                  frame No Error {
                  }
                  frame Error {
                    n440 = invoke class="VI" method="Ctrl Val.Get (Deprecated)"(reference=w914, error in=w915, "Control Name"="Base class") -> (reference out=w916:refnum<vi>, error out=w920:errorcluster, "Get Control Value"=w918:string)  [unwired: 2 in, 2 out]
                    n441 = case shown="Error" w920 {
                      selector: w920 -> [w923 _]
                      tunnel: [w923 w928] -> w919
                      tunnel: w918 -> [w922 _]
                      tunnel: [w922 w926] -> w917
                      tunnel: w916 -> [_ w931]
                      tunnel: w915 -> [_ w925]
                      frame No Error {
                      }
                      frame Error {
                        n442 = invoke class="VI" method="Ctrl Val.Get (Deprecated)"(reference=w931, error in=w925, "Control Name"="Data") -> (reference out=w924:refnum<vi>, error out=w929:errorcluster, "Get Control Value"=w927:string)  [unwired: 2 in, 2 out]
                        n443 = case shown="Error" w929 {
                          selector: w929 -> [w933 _]
                          tunnel: [w933 w937] -> w928
                          tunnel: w927 -> [w932 _]
                          tunnel: [w932 w936] -> w926
                          tunnel: w925 -> [_ w935]
                          tunnel: w924 -> [_ w934]
                          frame No Error {
                          }
                          frame Error {
                            n444 = invoke class="VI" method="Ctrl Val.Get (Deprecated)"(reference=w934, error in=w935, "Control Name"="Class attribute") -> (error out=w937:errorcluster, "Get Control Value"=w936:string)  [unwired: 2 in, 3 out]
                          }
                        }
                      }
                    }
                  }
                }
                n445 = Close Reference(reference=w882, error in (no error)=w883) -> ()  [unwired: 1 out]
                n446 = case shown="True" w901 {
                  tunnel: [_ w940] -> w900
                  tunnel: w897 -> [w939 w940]
                  tunnel: [w939 _] -> w899
                  frame False {
                  }
                  frame True {
                  }
                }
                n447 = call <resource>:"ProbeObjectKernel.vi"("ObjectStatus"=w911, "Ref"=w895, "ObjAttribute"=w899, "ClassAttribute"=w900, "ClassProvider"=w896, "error in"=w898, "Mode(Get)"=enum16{"Get", "Set", "Delete"}."Set") -> ("error out"=w902:errorcluster)  [unwired: 11 in, 1 out]
              }
            }
            n448 = Bundle By Name(cluster=w864, "CurrentClassViewing"=w862, "ClassAttributeViewing"=w861) -> (w863:T7)
          }
          frame "ShowAttribute" {
            n449 = Unbundle By Name(w959) -> ("ClassAttRefs"=w961:refnum<vi>[], "ClassAttribute"=w963:bool, "ObjRefs"=w962:refnum<vi>[])
            n450 = local read "_Classes"() -> (w953:u16)
            n451 = Decrement(x=w953) -> (x-1=w952:u16)
            n452 = Decrement(x=w952) -> (x-1=w951:u16)
            n453 = Select(t=w961, s=w963, f=w962) -> (s? t:f=w960:refnum<vi>[])
            n454 = Index Array(array=w960, index=w951) -> (element=w956:refnum<vi>)
            n455 = Not A Number/Path/Refnum?(number/path/refnum=w956) -> (NaN/Path/Refnum?=w958:bool)
            n456 = case shown="False" w958 {
              tunnel: w957 -> [w970 w971]
              tunnel: w956 -> [w967 _]
              tunnel: [w966 w971] -> w955
              frame False {
                n457 = invoke on="Attribute" class="SubPanel" method="Remove VI"(error in=w970) -> (error out=w965:errorcluster)  [unwired: 2 in, 2 out]
                n458 = property class="VI"(reference=w967, error in=w965, "Front Panel.Open"=FALSE ("Front Panel Window:Open")) -> (reference out=w964:refnum<vi>, error out=w968:errorcluster)
                n459 = invoke on="Attribute" class="SubPanel" method="Insert VI"(error in=w968, "VI Ref"=w964) -> (error out=w966:errorcluster)  [unwired: 2 in, 3 out]
              }
              frame True {
              }
            }
          }
          frame "KillObject" {
            n460 = local read "_Objects"() -> (w983:i32)
            n461 = Unbundle By Name(w984) -> ("ObjStatus"=w980:refnum<vi>[], "Classes"=w979:string[], "Objects"=w978:T9)
            n462 = call <vilib>:"Set Busy.vi"("error in (no error)"=w973) -> ("error out"=w972:errorcluster)  [unwired: 9 in, 1 out]
            n463 = Index Array(array=w978, index=w983) -> (element=w982:T12)
            n464 = case shown="0, Default" w983 {
              selector: w983 -> [w988 _]
              tunnel: w982 -> [w993 _]
              tunnel: w978 -> [w991 w995]
              tunnel: [w992 w995] -> w981
              tunnel: [w987 -1 ("Objects")] -> w977
              frame 0, Default {
                n465 = Array Size(array=w991) -> (size(s)=w990:i32)
                n466 = Build Array(w993) -> (w992:T9)
                n467 = Decrement(x=w990) -> (x-1=w989:i32)
                n468 = Decrement(x=w989) -> (x-1=w986:i32)
                n469 = Max & Min(x=w986, y=w988) -> (min(x,y)=w987:i32)  [unwired: 1 out]
              }
              frame -1 {
              }
            }
            n470 = local read "_NoOfObjects"() -> (w976:i32)
            n471 = local write "_Objects"(w977) -> ()
            n472 = for {
              shift-right: [w1008] -> w975
              shift-left: w972 -> [w1009]
              tunnel: w981 -> [w1005] mode=indexing
              tunnel: w980 -> [w1004]
              tunnel: w979 -> [w1001]
              tunnel: w976 -> [w1000]
              i -> [w999]
              n473 = Unbundle(w1005) -> ("Refs"=w1003:variant, "VI Name"=w1006:string, "ClassProvider"=w996:T3)  [unwired: 1 out]
              n474 = Increment(x=w999) -> (x+1=w998:i32)
              n475 = Subtract(x=w1000, y=w998) -> (x-y=w997:i32)
              n476 = Search 1D Array(1D array=w1001, element=w1006) -> (index of element=w1007:i32)  [unwired: 1 in]
              n477 = Index Array(array=w1004, index=w1007) -> (element=w1002:refnum<vi>)
              n478 = local write "_NoOfObjects"(w997) -> ()
              n479 = call <resource>:"ProbeObjectKernel.vi"("ObjectStatus"=w1002, "Ref"=w1003, "ClassProvider"=w996, "error in"=w1009, "Mode(Get)"=enum16{"Get", "Set", "Delete"}."Delete") -> ("error out"=w1008:errorcluster)  [unwired: 13 in, 1 out]
            }
            n480 = call <vilib>:"Unset Busy.vi"("error in (no error)"=w975) -> ("error out"=w974:errorcluster)  [unwired: 10 in]
          }
          frame "PrepareToModify" {
          }
          frame "CloseDown", "Error", Default {
            n481 = case shown="Default" w1016 {
              tunnel: ["Exit" "GetObjects"] -> w1018
              tunnel: w1017 -> [w1026 _]
              tunnel: w1015 -> [_ _]
              frame Default {
                n482 = Unbundle By Name(w1026) -> ("DebugQueue"=w1025:refnum<queue>, "ObjRefs"=w1021:refnum<vi>[], "ClassAttRefs"=w1022:refnum<vi>[], "ObjStatus"=w1023:refnum<vi>[], "MyComputerRef"=w1024:refnum<vi>, "ClRefs"=w1020:refnum<vi>[])  [unwired: 8 out]
                n483 = Close Reference(reference=w1020) -> ()  [unwired: 1 in, 1 out]
                n484 = Release Queue(queue=w1025) -> ()  [unwired: 2 in, 3 out]
                n485 = Close Reference(reference=w1021) -> ()  [unwired: 1 in, 1 out]
                n486 = Close Reference(reference=w1022) -> ()  [unwired: 1 in, 1 out]
                n487 = Close Reference(reference=w1024) -> ()  [unwired: 1 in, 1 out]
                n488 = Close Reference(reference=w1023) -> ()  [unwired: 1 in, 1 out]
                n489 = property on="_Objects" class="MCListbox (strict)"("ItemNames"=string[][] [] ("Item Names")) -> ()  [unwired: 2 in, 2 out]
              }
              frame "Error" {
              }
            }
          }
        }
        n490 = Equal?(x=w30, y="Exit") -> (x = y?=w34:bool)
        n491 = Select(t="Error", s=w28, f=w30) -> (s? t:f=w33:string)
      }
    }
    frame Error {
    }
  }
  "error out" <- w13
  n492 = call <resource>:"GDSError_ReportError.vi"("error in (no error)"=w13) -> ("error out"=w12:errorcluster)  [unwired: 18 in]
  n493 = stacked-sequence {
    tunnel: w12 -> [_]
    tunnel: w9 -> [w1031]
    frame #0 {
      n494 = property class="VI"() -> ("Front Panel.WinBounds"=w1035:T5, "FP.Behavior"=w1034:T8)  [unwired: 2 in, 2 out]
      n495 = Bundle("Front Panel.WinBounds"=w1035, "FP.Behavior"=w1034) -> (w1033:T6)  [unwired: 1 in]
      n496 = Flatten To XML(6:w1033) -> (2:w1032:string)
      n497 = Write to Text File(file (use dialog)=w1031, text=w1032) -> (error out=w1030:errorcluster)  [unwired: 2 in, 2 out]
      n498 = stacked-sequence {
        tunnel: w1030 -> [_]
        frame #0 {
          n499 = property class="VI"("Front Panel.Open"=FALSE ("Front Panel Window:Open")) -> ()  [unwired: 2 in, 2 out]
        }
      }
    }
  }
